vi "PressureSensor.vi"(7 "Action":T4, 8 "error in (no error)":errorcluster, 11 "AIDeviceRef":T1={"DevStatus"={"status"=FALSE, "code"=0, "source"=""}, "Analog Module"=enum."Analog Module 1", "Analog Channel"=enum."Invalid"}) -> (0 "error out":errorcluster, 3 "Pressure":dbl)   [LabVIEW 2013]
doc: "Reads the pressure from the pressure sensor. It has the following actions:\n-Init: takes a reference to an analog channel and stores it.\n-ReadValue: uses a linear fit to return the pressure based on the voltage read from the analog channel.\n-Disable: no action."
uses:
  Example_Code/PressureSensor/PressureSensorAction.ctl
  <vilib>/Rock Robotics/WPI/AnalogChannel/WPI_AnalogChannelDevRef.ctl
  <vilib>/Rock Robotics/SystemInterfaces/Typedef/FPGA_TypedefAnalogModule.ctl
  <vilib>/Rock Robotics/SystemInterfaces/AI/FPGA_AIChannel.ctl
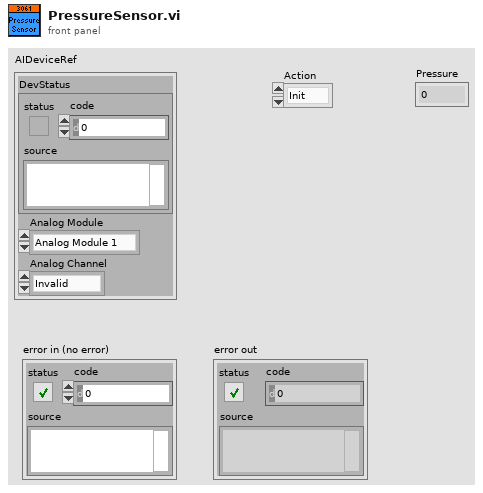
[diagram p1: front panel]
types:
  T1 = typedef "WPI_AnalogChannelDevRef.ctl" = cluster{"DevStatus":errorcluster, "Analog Module":T2, "Analog Channel":T3}
  T2 = typedef "FPGA_TypedefAnalogModule.ctl" = enum16{"Analog Module 1", "Analog Module 2"}
  T3 = typedef "FPGA_AIChannel.ctl" = enum8{"AI 1", "AI 2", "AI 3", "AI 4", "AI 5", "AI 6", "AI 7", "AI 8", "Invalid"}
  T4 = typedef "PressureSensorAction.ctl" = enum16{"Init", "ReadValue", "Disable"}
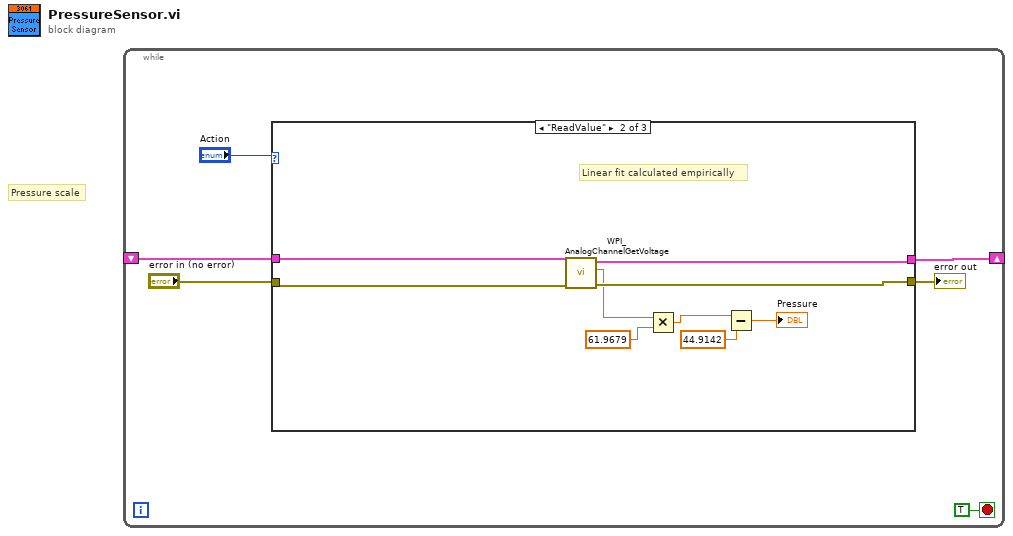
[diagram p0: block diagram]
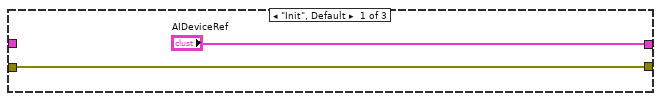
[diagram p2: hidden frame]
diagram:
  # "Pressure scale"
  n1 = while {
    shift-right: [w5] -> _
    shift-left: _ -> [w4]
    stop <- TRUE stop-if-true
    n2 = case shown="\"ReadValue\"" "Action" {
      tunnel: ["AIDeviceRef" w16 w19] -> w5
      tunnel: w4 -> [_ w17 w19]
      tunnel: "error in (no error)" -> [w7 w15 w18]
      tunnel: [w7 w14 w18] -> w2
      frame "Init", Default {
      }
      frame "ReadValue" {
        # "Linear fit calculated empirically"
        n3 = call <vilib>:"WPI_AnalogChannelGetVoltage.vi"("error in (no error)"=w15, "AIDeviceRef"=w17) -> ("error out"=w14:errorcluster, "Voltage"=w12:dbl, "AIDeviceRef"=w16:T1)  [unwired: 7 in]
        n4 = Multiply(x=w12, y=61.9679 ("x")) -> (x*y=w10:dbl)
        n5 = Subtract(x=w10, y=44.9142 ("x")) -> (x-y=→"Pressure":dbl)
      }
      frame "Disable" {
      }
    }
    "error out" <- w2
  }
